vi "MTS_BuildWSTree.vi"(7 "Action":enum16{"Rebuild Tree", "Add to Tree"}(ring), 8 "error in":errorcluster, 10 "Files in Workspace":T1(array[cluster]), 11 "Tree Refnum":refnum<vi>) -> (0 "error out":errorcluster, 3 "Tree Refnum (dup)":refnum<vi>)   [LabVIEW 2010]
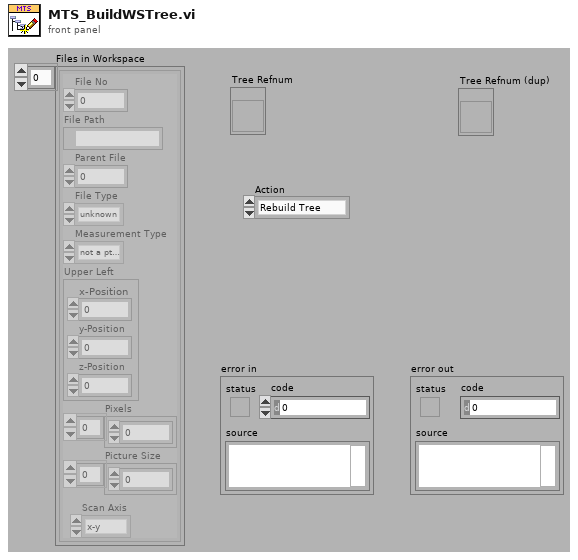
[diagram p1: front panel]
types:
  T1 = cluster{"File No":i32, "File Path":path, "Parent File":i32, "File Type":enum16{"unknown", "pt3 File", "png Image", "bmp Image"}, "Measurement Type":enum16{"not a pt3 File", "Image File", "Point Measurement", "Auto Point"}, "Upper Left":cluster{"x-Position":dbl, "y-Position":dbl, "z-Position":dbl}, "Pixels":i32[], "Picture Size":dbl[], "Scan Axis":enum32{"x-y", "x-z", "y-z"}}[]
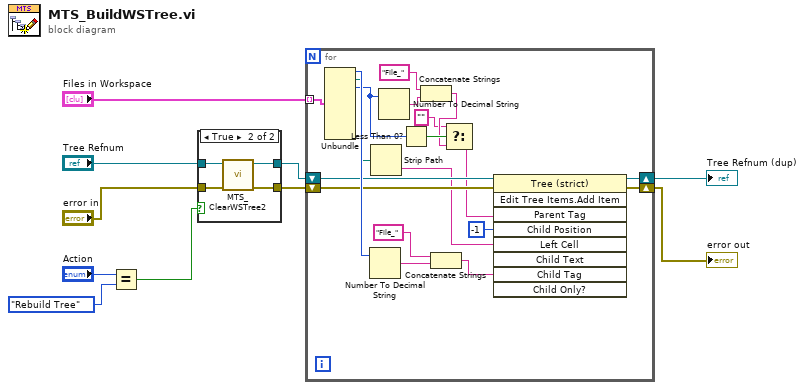
[diagram p0: block diagram]
diagram:
  n1 = Equal?(x="Action", y=enum16{"Rebuild Tree", "Add to Tree"}."Rebuild Tree") -> (x = y?=w1:bool)
  n2 = case shown="True" w1 {
    tunnel: "Tree Refnum" -> [w12 w16]
    tunnel: "error in" -> [w11 w15]
    tunnel: [w11 w14] -> w7
    tunnel: [w12 w13] -> w6
    frame False {
    }
    frame True {
      n3 = call "MTS_ClearWSTree2.vi"("error in"=w15, "Tree Refnum"=w16) -> ("error out"=w14:errorcluster, "Tree Refnum (dup)"=w13:refnum<vi>)  [unwired: 8 in]
    }
  }
  n4 = for {
    tunnel: "Files in Workspace" -> [w35] mode=indexing
    shift-right: [w29] -> w4
    shift-left: w7 -> [w31]
    shift-right: [w28] -> w5
    shift-left: w6 -> [w30]
    n5 = Unbundle(w35) -> ("File No"=w34:i32, "File Path"=w20:path, "Parent File"=w26:i32)  [unwired: 6 out]
    n6 = Number To Decimal String(number=w34) -> (decimal integer string=w33:string)  [unwired: 1 in]
    n7 = Strip Path(path=w20) -> (name=w19:string)  [unwired: 1 out]
    n8 = Number To Decimal String(number=w26) -> (decimal integer string=w25:string)  [unwired: 1 in]
    n9 = Less Than 0?(x=w26) -> (x < 0?=w27:bool)
    n10 = Concatenate Strings("File_" ("decimal integer string"), w25) -> (w23:string)
    n11 = Concatenate Strings("File_" ("decimal integer string"), w33) -> (w18:string)
    n12 = Select(t="", s=w27, f=w23) -> (s? t:f=w21:string)
    n13 = invoke on="Invoke Node" class="Tree (strict)" method="Edit Tree Items.Add Item"(reference=w30, error in=w31, "Parent Tag"=w21, "Child Position"=-1, "Left Cell"=w19, "Child Tag"=w18) -> (reference out=w28:refnum<vi>, error out=w29:errorcluster)  [unwired: 3 in, 7 out]
  }
  "error out" <- w4
  "Tree Refnum (dup)" <- w5
